vi "HEWH RLT GET Flow Data.vi"(6 "Collect Power Data":bool, 8 "Error In":errorcluster, 10 "All Other Data (NO TC's) in":string[][](array[string])) -> (0 "Error Out":errorcluster, 3 "All Other Data (NO TC's) out":string[][](array[string]))   [LabVIEW 2023]
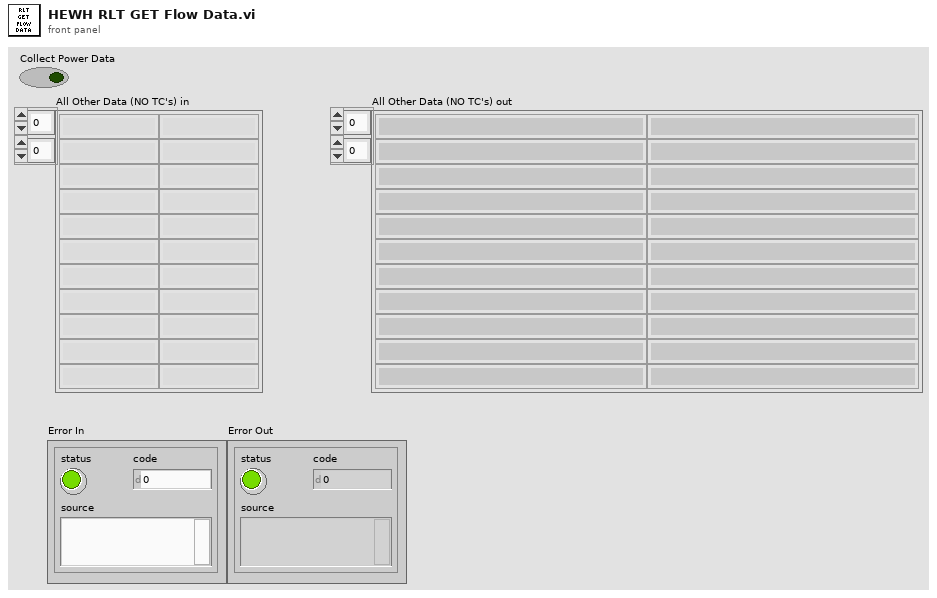
[diagram p1: front panel]
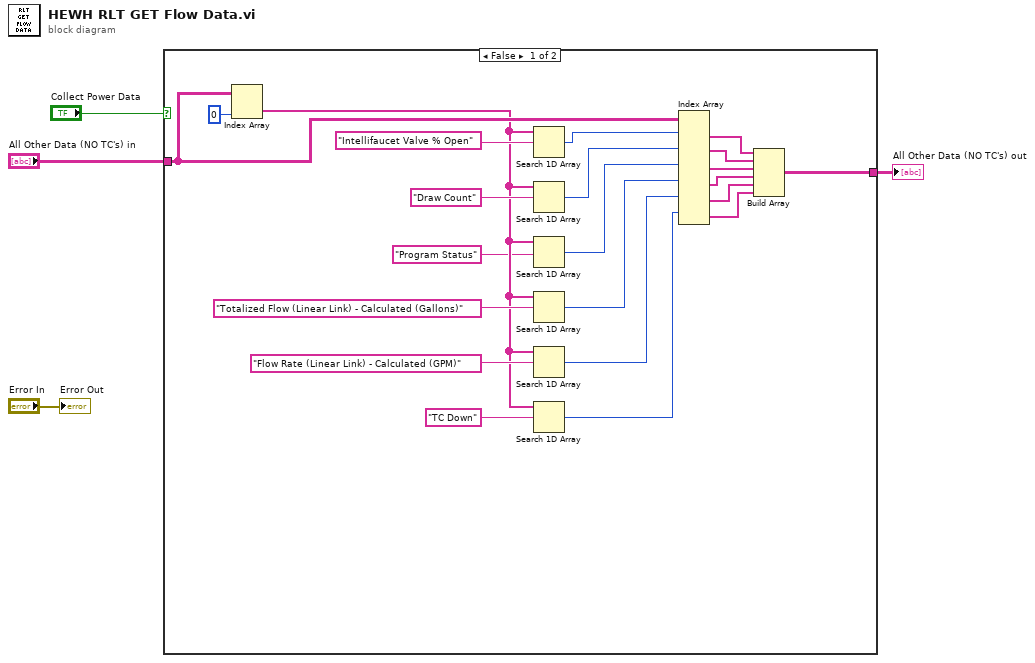
[diagram p0: block diagram]
diagram:
  n1 = case shown="False" "Collect Power Data" {
    tunnel: [w15 w27] -> w2
    tunnel: "All Other Data (NO TC's) in" -> [w20 w27]
    frame False {
      n2 = Index Array(array=w20, index (col)=0 ("disabled index (col)")) -> (element=w7:string[])  [unwired: 1 in]
      n3 = Search 1D Array(1D array=w7, element="Intellifaucet Valve % Open") -> (index of element=w19:i32)  [unwired: 1 in]
      n4 = Search 1D Array(1D array=w7, element="Draw Count") -> (index of element=w18:i32)  [unwired: 1 in]
      n5 = Search 1D Array(1D array=w7, element="Program Status") -> (index of element=w8:i32)  [unwired: 1 in]
      n6 = Search 1D Array(1D array=w7, element="Totalized Flow (Linear Link) - Calculated (Gallons)") -> (index of element=w12:i32)  [unwired: 1 in]
      n7 = Search 1D Array(1D array=w7, element="Flow Rate (Linear Link) - Calculated (GPM)") -> (index of element=w13:i32)  [unwired: 1 in]
      n8 = Search 1D Array(1D array=w7, element="TC Down") -> (index of element=w14:i32)  [unwired: 1 in]
      n9 = Index Array(array=w20, index (row) #1=w19, index (row) #2=w18, index (row) #3=w8, index (row) #4=w12, index (row) #5=w13, index (row) #6=w14) -> (element #1=w17:string[], element #2=w16:string[], element #3=w5:string[], element #4=w9:string[], element #5=w10:string[], element #6=w11:string[])  [unwired: 6 in]
      n10 = Build Array(w17, w16, w5, w9, w10, w11) -> (w15:string[][])
    }
    frame True {
    }
  }
  "All Other Data (NO TC's) out" <- w2
  "Error Out" <- "Error In"
